vi "ReadErrInfo.vi"(8 "Error In(No Error)":errorcluster, 11 "CAN Device In":T1={"Device Type"=20, "Device Index"=0, "CANInd"=0, "Baud(E_U)"=1835016} {"Baud(E_U)" items=["1000Kbps"=393219, "800Kbps"=393220, "500Kbps"=393223, "250Kbps"=1835016, "125Kbps"=1835025, "100Kbps"=1441827, "50Kbps"=1835052, "20Kbps"=1441971, "10Kbps"=1835232, "5Kbps"=1835457]; "Device Type" items=["PCI5121"=1, "PCI9810"=2, "USBCAN1"=3, "USBCAN2"=4, "PCI9820"=5, "PCI5110"=7, "PC104CAN"=11, "CANETUDP"=12, "PCI9840B"=14, "PC104C2"=15, "PCI9820I"=16, "CANETTCP"=17, "PCIE9221"=24, "PCI5010U"=19, "USBCAN_E_U"=20, "USBCAN_2E_U"=21, "PCI5020U"=22, "PCIE9120I"=27, "PCIE9110I"=28, "PCIE9140I"=29, "USBCAN-4E-U"=31, "USBCAN-8E-U"=34]}) -> (0 "Error Out":errorcluster, 2 "VCI_ERR_INFO":T2, 3 "CAN Device Out":T1={"Device Type"=20, "Device Index"=0, "CANInd"=0, "Baud(E_U)"=1835016} {"Baud(E_U)" items=["1000Kbps"=393219, "800Kbps"=393220, "500Kbps"=393223, "250Kbps"=1835016, "125Kbps"=1835025, "100Kbps"=1441827, "50Kbps"=1835052, "20Kbps"=1441971, "10Kbps"=1835232, "5Kbps"=1835457]; "Device Type" items=["PCI5121"=1, "PCI9810"=2, "USBCAN1"=3, "USBCAN2"=4, "PCI9820"=5, "PCI5110"=7, "PC104CAN"=11, "CANETUDP"=12, "PCI9840B"=14, "PC104C2"=15, "PCI9820I"=16, "CANETTCP"=17, "PCIE9221"=24, "PCI5010U"=19, "USBCAN_E_U"=20, "USBCAN_2E_U"=21, "PCI5020U"=22, "PCIE9120I"=27, "PCIE9110I"=28, "PCIE9140I"=29, "USBCAN-4E-U"=31, "USBCAN-8E-U"=34]})   [LabVIEW 2020, in "ZLGCAN.lvclass"]
uses:
  ZLGCAN.lvclass
  Device.ctl
  ControlCAN.dll
panel:
  out "return type":u32
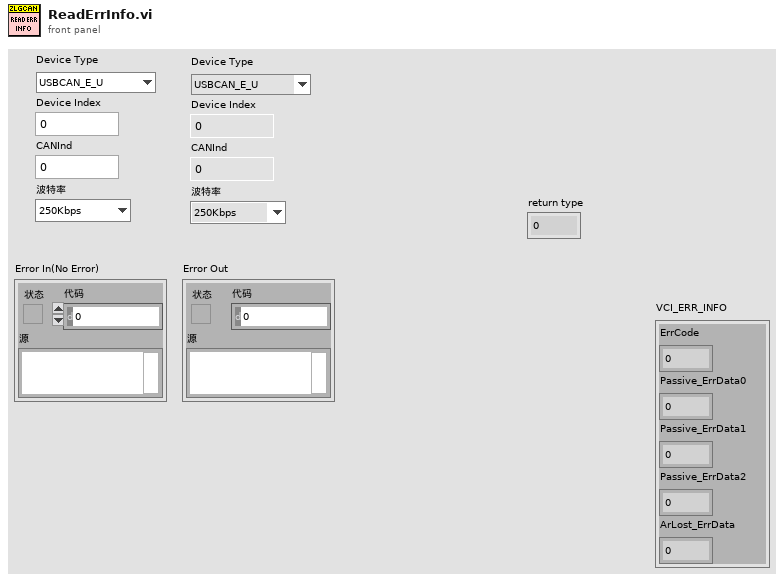
[diagram p1: front panel]
types:
  T1 = typedef "ZLGCAN.lvclass/Device.ctl" = cluster{"Device Type":u32, "Device Index":u32, "CANInd":u32, "Baud(E_U)":u32}
  T2 = cluster{"ErrCode":u32, "Passive_ErrData0":u8, "Passive_ErrData1":u8, "Passive_ErrData2":u8, "ArLost_ErrData":u8}
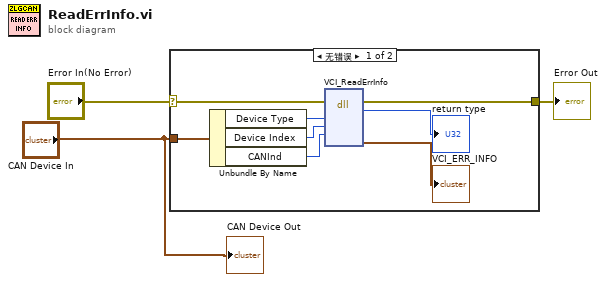
[diagram p0: block diagram]
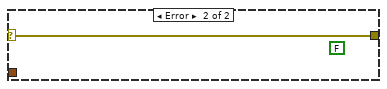
[diagram p2: hidden frame]
diagram:
  n1 = case shown="无错误" "Error In(No Error)" {
    selector: "Error In(No Error)" -> [w10 w12]
    tunnel: [w4 w12] -> w2
    tunnel: "CAN Device In" -> [w9 _]
    frame No Error {
      n2 = Unbundle By Name(w9) -> ("Device Type"=w8:u32, "Device Index"=w7:u32, "CANInd"=w6:u32)
      n3 = dll-call lib="PTH2sabs CUsersxu.dongDesktop新建文件夹新建文件夹 (2) - 副本ZLGCAN\nControlCANControlCAN.dll" fn="VCI_ReadErrInfo"(error in=w10, "DeviceType"=w8, "DeviceInd"=w7, "CANInd"=w6) -> (error out=w4:errorcluster, "返回类型"=→"return type":u32, "VCI_ERR_INFO"=→"VCI_ERR_INFO":T2)  [unwired: 5 in, 2 out]
    }
    frame Error {
      (unwired) FALSE
    }
  }
  "Error Out" <- w2
  "CAN Device Out" <- "CAN Device In"
